vi "svx_Crop X to scale.vi"(7 "Display State In":T1={"X Scale Width %"=50.0, "Y Scale Height %"=50.0, "X-Axis Range"={"Minimum"=0.0, "Maximum"=10.0}, "Y-Axis Range"={"Minimum"=0.0, "Maximum"=10.0}, "Z-Axis Range"={"Minimum"=0.0, "Maximum"=10.0}, "Plot Color"=61212, "Frame Color"=16252785, "Background Color"=16777222, "Initial AutoScale Y"=TRUE, "AutoScale X"=2, "AutoScale Y"=2, "AutoScale Z"=2, "Plot Transparency"=FALSE, "X-Axis Name"="Frequency", "Y-Axis Name"="Amplitude", "Z-Axis Name"="", "X-Axis Scaling Factor"={"Offset"=0.0, "Multiplier"=1.0}, "Y-Axis Scaling Factor"={"Offset"=0.0, "Multiplier"=1.0}, "Z-Axis Scaling Factor"={"Offset"=0.0, "Multiplier"=1.0}, "X-Scale Visible"=TRUE, "Y-Scale Visible"=TRUE, "Z-Scale Visible"=TRUE, "X-Scale Label Visible"=TRUE, "Y-Scale Label Visible"=TRUE, "Z-Scale Label Visible"=TRUE, "X-Axis Range Scaled"={"Minimum"=0.0, "Maximum"=10.0}, "Y-Axis Range Scaled"={"Minimum"=0.0, "Maximum"=10.0}, "Z-Axis Range Scaled"={"Minimum"=0.0, "Maximum"=10.0}, "Rev Z Order"=FALSE, "X-Scale Format Str"="%#.4g", "Y-Scale Format Str"="%#.4g", "Z-Scale Format Str"="%#.4g", "Decor color"=12369084, "Scale Range Change"=refnum, "out of state queue"=refnum, "property nodes"=refnum, "Lines"=[], "Line Properties"={"Line Color"=61212, "Line Width"=61212, "Line Style"=enum."Dash", "DisplayLines"=FALSE}} caption="State" {"Line Properties"."Line Width" min=1}, 9 "Cropped Info":cluster{"First Index":i32, "Length":i32}, 11 "Plots":cluster{"x0":dbl, "dx":dbl, "Y":dbl[]}[](array[cluster])) -> (1 "Cropped Info out":cluster{"First Index":i32, "Length":i32}, 3 "Plots":cluster{"x0":dbl, "dx":dbl, "Y":dbl[]}[](array[cluster]))   [LabVIEW 2017, in "SVX Waterfall Graph.xctl"]
uses:
  <vilib>/addons/_XControls/Waterfall Graph/SVX Waterfall Graph.xctl
  <vilib>/addons/_XControls/Waterfall Graph/subVIs/svx_Waterfall State.ctl
  <vilib>/addons/_NISVFA/_Shared subVIs/Controls/svc_Cluster of Array of Cluster of XYZ.ctl
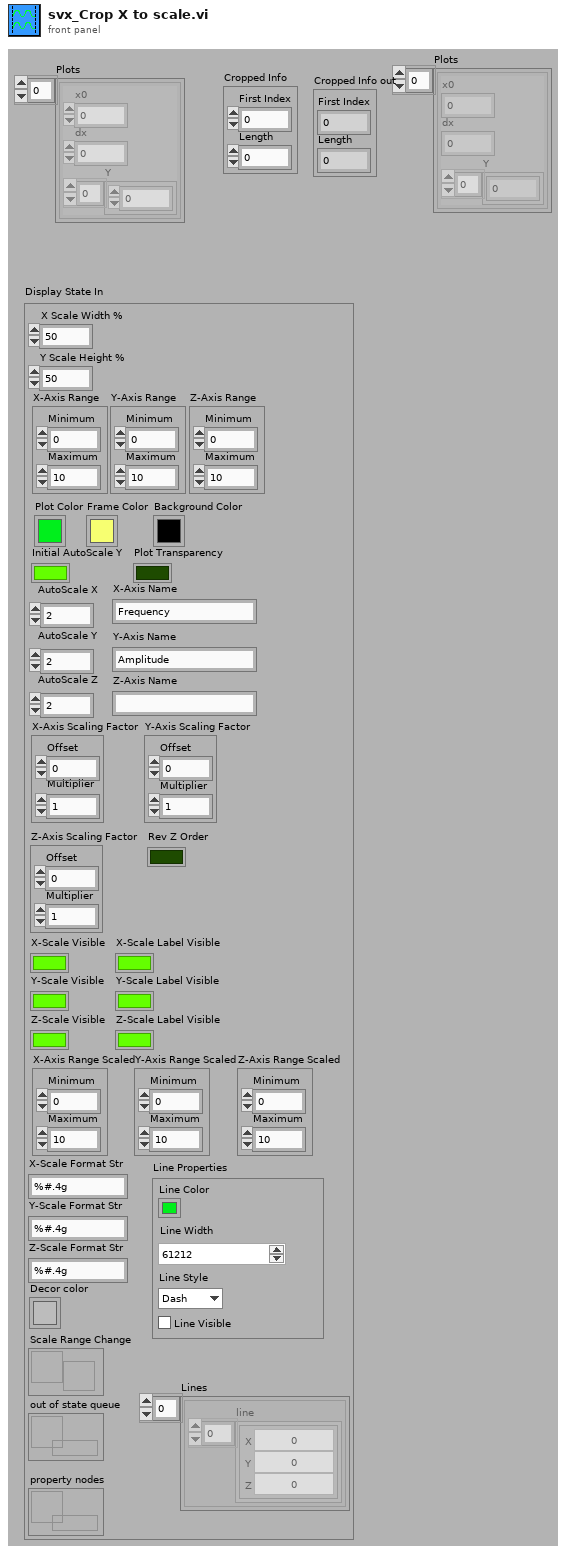
[diagram p1: front panel]
types:
  T1 = typedef "SVX Waterfall Graph.xctl/svx_Waterfall State.ctl" = cluster{"X Scale Width %":dbl, "Y Scale Height %":dbl, "X-Axis Range":cluster{"Minimum":dbl, "Maximum":dbl}, "Y-Axis Range":cluster{"Minimum":dbl, "Maximum":dbl}, "Z-Axis Range":cluster{"Minimum":dbl, "Maximum":dbl}, "Plot Color":u32, "Frame Color":u32, "Background Color":u32, "Initial AutoScale Y":bool, "AutoScale X":u8, "AutoScale Y":u8, "AutoScale Z":u8, "Plot Transparency":bool, "X-Axis Name":string, "Y-Axis Name":string, "Z-Axis Name":string, "X-Axis Scaling Factor":cluster{"Offset":dbl, "Multiplier":dbl}, "Y-Axis Scaling Factor":cluster{"Offset":dbl, "Multiplier":dbl}, "Z-Axis Scaling Factor":cluster{"Offset":dbl, "Multiplier":dbl}, "X-Scale Visible":bool, "Y-Scale Visible":bool, "Z-Scale Visible":bool, "X-Scale Label Visible":bool, "Y-Scale Label Visible":bool, "Z-Scale Label Visible":bool, "X-Axis Range Scaled":cluster{"Minimum":dbl, "Maximum":dbl}, "Y-Axis Range Scaled":cluster{"Minimum":dbl, "Maximum":dbl}, "Z-Axis Range Scaled":cluster{"Minimum":dbl, "Maximum":dbl}, "Rev Z Order":bool, "X-Scale Format Str":string, "Y-Scale Format Str":string, "Z-Scale Format Str":string, "Decor color":u32, "Scale Range Change":refnum<user-event>, "out of state queue":refnum<queue>, "property nodes":refnum<queue>, "Lines":T2[], "Line Properties":cluster{"Line Color":u32, "Line Width":u16, "Line Style":enum32{"Solid", "Dash", "Dot", "DashDot", "DashDotDot"}, "DisplayLines":bool}}
  T2 = typedef "svc_Cluster of Array of Cluster of XYZ.ctl" = cluster{"line":cluster{"X":dbl, "Y":dbl, "Z":dbl}[]}
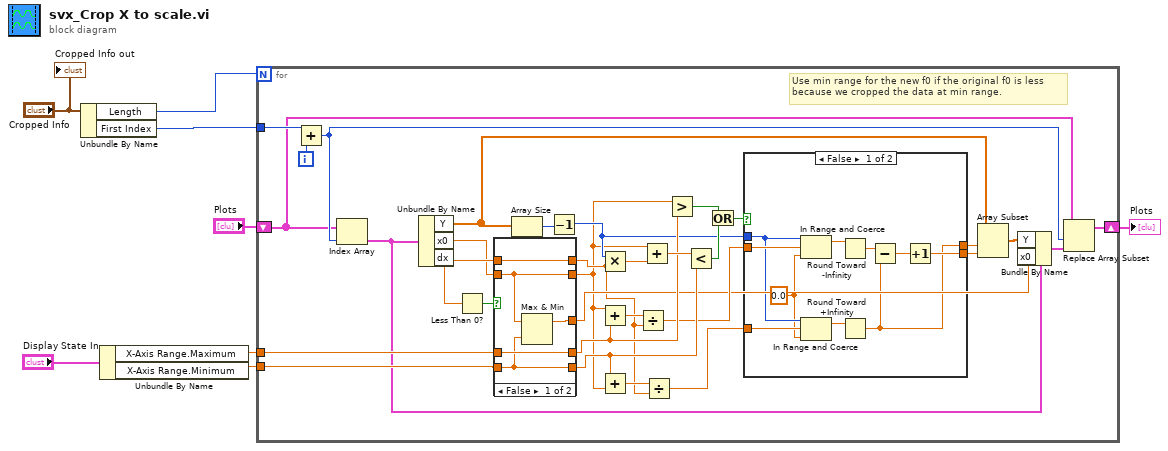
[diagram p0: block diagram]
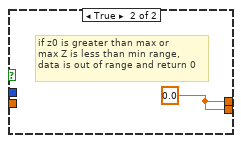
[diagram p2: hidden frame]
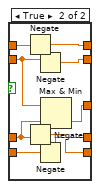
[diagram p3: hidden frame]
diagram:
  n1 = Unbundle By Name("Cropped Info") -> ("Length"=w8:i32, "First Index"=w7:i32)
  n2 = Unbundle By Name("Display State In") -> ("X-Axis Range.Maximum"=w2:dbl, "X-Axis Range.Minimum"=w3:dbl)
  n3 = for {
    N: w8 -> [_]
    tunnel: w2 -> [w39]
    tunnel: w3 -> [w38]
    tunnel: w7 -> [w13]
    shift-right: [w9] -> w4
    shift-left: "Plots" -> [w10]
    i -> [w14]
    # "Use min range for the new f0 if the original f0 is less \nbecause we cropped the data at min range."
    n4 = Add(x=w13, y=w14) -> (x+y=w12:i32)
    n5 = Index Array(array=w10, index=w12) -> (element=w15:cluster{"x0":dbl, "dx":dbl, "Y":dbl[]})
    n6 = Unbundle By Name(w15) -> ("Y"=w21:dbl[], "x0"=w36:dbl, "dx"=w40:dbl)
    n7 = Less Than 0?(x=w40) -> (x < 0?=w37:bool)
    n8 = case shown="False" w37 {
      tunnel: w40 -> [w56 w65]
      tunnel: [w56 w64] -> w17
      tunnel: w36 -> [w53 w58]
      tunnel: [w53 w63] -> w16
      tunnel: w39 -> [w55 w59]
      tunnel: w38 -> [w54 w62]
      tunnel: [w55 w61] -> w27
      tunnel: [w54 w60] -> w28
      tunnel: [w52 w57] -> w22
      frame False {
        n9 = Max & Min(x=w53, y=w54) -> (max(x,y)=w52:dbl)  [unwired: 1 out]
      }
      frame True {
        n10 = Negate(x=w65) -> (-x=w64:dbl)
        n11 = Negate(x=w59) -> (-x=w60:dbl)
        n12 = Negate(x=w58) -> (-x=w63:dbl)
        n13 = Negate(x=w62) -> (-x=w61:dbl)
        n14 = Max & Min(x=w58, y=w59) -> (min(x,y)=w57:dbl)  [unwired: 1 out]
      }
    }
    n15 = Array Size(array=w21) -> (size(s)=w29:i32)
    n16 = Decrement(x=w29) -> (x-1=w24:i32)
    n17 = Multiply(x=w24, y=w17) -> (x*y=w33:dbl)
    n18 = Add(x=w16, y=w27) -> (x+y=w34:dbl)
    n19 = Add(x=w28, y=w16) -> (x+y=w35:dbl)
    n20 = Divide(x=w34, y=w17) -> (x/y=w25:dbl)
    n21 = Add(x=w16, y=w33) -> (x+y=w30:dbl)
    n22 = Divide(x=w35, y=w17) -> (x/y=w26:dbl)
    n23 = Greater?(x=w16, y=w27) -> (0:w31:bool)
    n24 = Less?(x=w30, y=w28) -> (x < y?=w32:bool)
    n25 = Or(x=w31, y=w32) -> (x .or. y?=w23:bool)
    n26 = case shown="False" w23 {
      tunnel: w25 -> [w47 _]
      tunnel: w26 -> [w46 _]
      tunnel: w24 -> [w44 _]
      tunnel: [w42 w51] -> w20
      tunnel: [w41 w51] -> w19
      frame False {
        w43 = 0.0 ("lower limit")
        n27 = In Range and Coerce(upper limit=w44, x=w47, lower limit=w43) -> (coerced(x)=w48:dbl)  [unwired: 1 out]
        n28 = In Range and Coerce(upper limit=w44, x=w46, lower limit=w43) -> (coerced(x)=w45:dbl)  [unwired: 1 out]
        n29 = Round Toward -Infinity(1:w48) -> (0:w50:dbl)
        n30 = Round Toward +Infinity(x=w45) -> (ceil(x): smallest int >= x=w41:dbl)
        n31 = Subtract(x=w50, y=w41) -> (x-y=w49:dbl)
        n32 = Increment(x=w49) -> (x+1=w42:dbl)
      }
      frame True {
        w51 = 0.0
        # "if z0 is greater than max or\nmax Z is less than min range,\ndata is out of range and return 0"
      }
    }
    n33 = Array Subset(array=w21, index=w19, length=w20) -> (w18:dbl[])
    n34 = Bundle By Name(cluster=w15, "Y"=w18, "x0"=w22) -> (w11:cluster{"x0":dbl, "dx":dbl, "Y":dbl[]})
    n35 = Replace Array Subset(array=w10, new element=w11, index=w12) -> (w9:cluster{"x0":dbl, "dx":dbl, "Y":dbl[]}[])
  }
  "Plots" <- w4
  "Cropped Info out" <- "Cropped Info"
